vi "Initialize File IO Loop.vi"(8 "error in":errorcluster, 11 "File Loop Data in":T1) -> (0 "error out":errorcluster, 3 "File Loop Data out":T1)   [LabVIEW 2018]
doc: "Reads in the file path for stored data, initializes the SR list by reading from SR list.txt, and sets the file path"
uses:
  Type Defs/File IO Loop Data.ctl
  Support/Message Queue/Message Cluster.ctl
  Type Defs/FGV States.ctl
  Support/Message Queue/Message Queue.lvlib
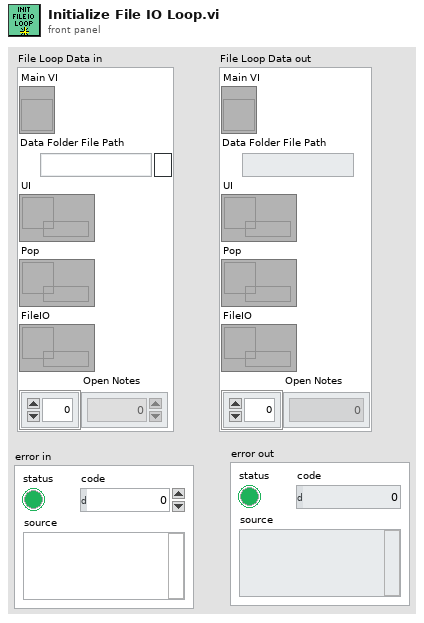
[diagram p1: front panel]
types:
  T1 = typedef "File IO Loop Data.ctl" = cluster{"Main VI":refnum<vi>, "Data Folder File Path":path, "UI":refnum<queue>, "Pop":refnum<queue>, "FileIO":refnum<queue>, "Open Notes":i32[]}
  T2 = typedef "FGV States.ctl" = enum16{"Initialize", "Merge", "Write", "Remove", "Read", "Clear"}
  T3 = typedef "SR Cluster.ctl" = cluster{"Color":u32, "SR Number":i32, "SR Status":T4, "Name":string, "Summary":string, "Last Updated":timestamp, "SR Type":string, "Service Level":string, "Days Open":dbl, "Creation Date":timestamp, "Owner":string, "Note":string}
  T4 = typedef "SR Status.ctl" = enum16{"Caller Abandoned", "Created in Error", "Expired", "Forum Resolved AE", "Forum Resolved Customer", "IN WORK", "IN WORK Collab with AES", "IN WORK Collab with PSE", "IN WORK Collab with SE", "IN WORK Customer Added Note", "IN WORK Escalation", "IN WORK Wait on Customer", "Open", "Potentially Resolved", "Presumed Resolved", "RMA Approved for Return", "RMA Closed", "RMA Closed - DOA", "RMA In Progress", "RMA Open", "RMA Waiting on Customer", "Resolved", "Passed Off"}
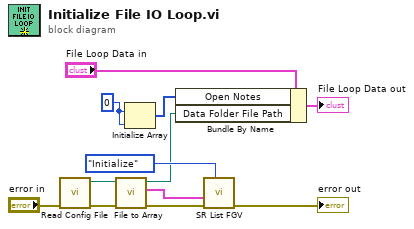
[diagram p0: block diagram]
diagram:
  w2 = 0 ("dimension size")
  n1 = call "Read Config File.vi"("error in (no error)"="error in") -> ("error out"=w6:errorcluster, "Data Folder Path"=w5:path)  [unwired: 7 in, 2 out]
  n2 = call "File to Array.vi"("error in"=w6, "file path in"=w5) -> ("error out"=w10:errorcluster, "list out"=w11:T3[], "file path out"=w4:path)  [unwired: 7 in]
  n3 = Initialize Array(w2, w2) -> (w1:i32[])
  n4 = Bundle By Name(cluster="File Loop Data in", "Open Notes"=w1, "Data Folder File Path"=w4) -> (→"File Loop Data out":T1)
  n5 = call "SR List FGV.vi"("Operation"=FGV_States."Initialize", "Error In"=w10, "Input"=w11) -> ("Error Out"=→"error out":errorcluster)  [unwired: 7 in, 1 out]
